vi "Get Timing.vi"(11 "Plugin Configuration in":refnum<class "Plugin Configuration.lvclass">) -> (2 "cycle timing":T1={"priority"=0, "decimation"=1, "offset"=0}, 3 "Plugin Configuration out":refnum<class "Plugin Configuration.lvclass">)   [LabVIEW 2017, in "Data Sharing Framework Engine.lvlib" / "Plugin Configuration.lvclass"]
uses:
  Plugin Configuration.lvclass
  old/dsf core/Source/DSF Configuration API/1.0.0/Public/Controls/DSF Timing Info.ctl
  Plugin Configuration.lvclass/Plugin Configuration.ctl
  old/dsf core/Source/DSF Configuration API/1.0.0/DSF Configuration API.lvlib
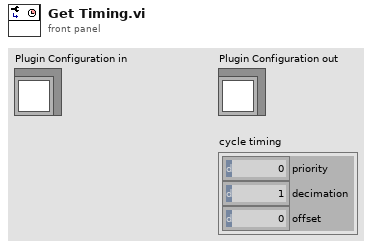
[diagram p1: front panel]
types:
  T1 = typedef "DSF Configuration API.lvlib/DSF Timing Info.ctl" = cluster{"priority":u64, "decimation":u64, "offset":u64}
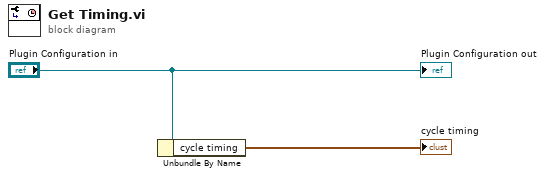
[diagram p0: block diagram]
diagram:
  n1 = Unbundle By Name("Plugin Configuration in") -> ("cycle timing"=→"cycle timing":T1)
  "Plugin Configuration out" <- "Plugin Configuration in"
